vi "Select Personality.vi"(8 "error in (no error)":errorcluster, 10 "Personality (0: Spectrum Analyzer)":u16(ring) items=["Spectrum Analyzer", "Phase Noise", "Noise Figure"], 11 "VISA resource name":refnum<visa-resource-name>) -> (0 "error out":errorcluster, 3 "VISA resource name out":refnum<visa-resource-name>)   [LabVIEW 2014, in "Agilent ESA PSA Series.lvlib"]
doc: "Selects the personality to be used for measurements. Use this VI to switch to different personalities required by other VIs.\n\n<B>Note:</B> \n\nSome personalities require additional hardware and/or software, installed on the analyzer.\n\nIf your VI's are failing because switching personalities are taking longer than the delay defined on the block diagram, try increasing the wait time to accomodate."
uses:
  Agilent ESA PSA Series.lvlib
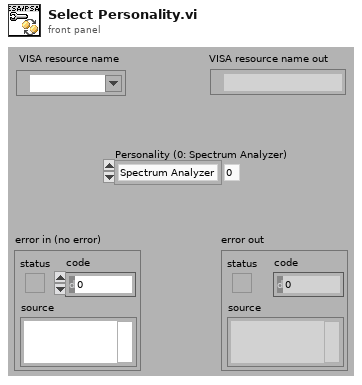
[diagram p1: front panel]
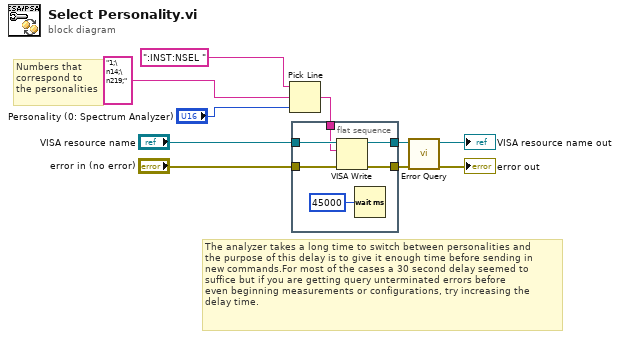
[diagram p0: block diagram]
diagram:
  # "Numbers that\ncorrespond to\nthe personalities"
  # "The analyzer takes a long time to switch between personalities and\nthe purpose of this delay is to give it enough time before sending in\nnew commands.For most of the cases a 30 second delay seemed to\nsuffice but if you are getting query unterminated errors before\neven beginning measurements or configurations, try increasing the\ndelay time."
  n1 = Pick Line(string ("")=":INST:NSEL ", multi-line string="1;\n14;\n219;", line index="Personality (0: Spectrum Analyzer)") -> (output string=w4:string)
  n2 = flat-sequence {
    tunnel: [w16] -> w10
    tunnel: [w15] -> w8
    tunnel: "VISA resource name" -> [w14]
    tunnel: "error in (no error)" -> [w13]
    tunnel: w4 -> [w12]
    frame #0 {
      n3 = VISA Write(VISA resource name=w14, write buffer=w12, error in (no error)=w13) -> (VISA resource name out=w16:refnum<visa-resource-name>, error out=w15:errorcluster)  [unwired: 1 out]
      n4 = Wait (ms)(milliseconds to wait=u32 45000) -> ()  [unwired: 1 out]
    }
  }
  n5 = call "Error Query.vi"("error in (no error)"=w8, "VISA resource name"=w10) -> ("error out"=→"error out":errorcluster, "VISA resource name out"=→"VISA resource name out":refnum<visa-resource-name>)  [unwired: 6 in, 2 out]
